vi "Check input.vi"(2 "String to check for":string, 3 "Old table to replace":string[][](table)=[["1", " "], ["2", " "], ["3", " "], ["4", " "], ["5", " "], ["6", " "], ["7", " "], ["8", " "], ["9", " "]]) -> (0 "Guess is correct?":bool, 1 "Output table":string[][](table)=[["1", " "], ["2", " "], ["3", " "], ["4", " "], ["5", " "], ["6", " "], ["7", " "], ["8", " "], ["9", " "]])   [LabVIEW 2023]
panel:
  in  "Answer array":string[](array[string])=["Bulbasaur", "Ivysaur", "Venusaur", "Charmander", "Charmeleon", "Charizard", "Squirtle", "Wartortle", "Blastoise"]
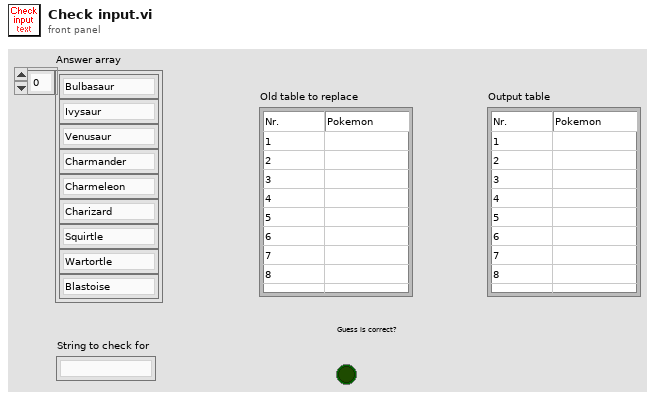
[diagram p1: front panel]
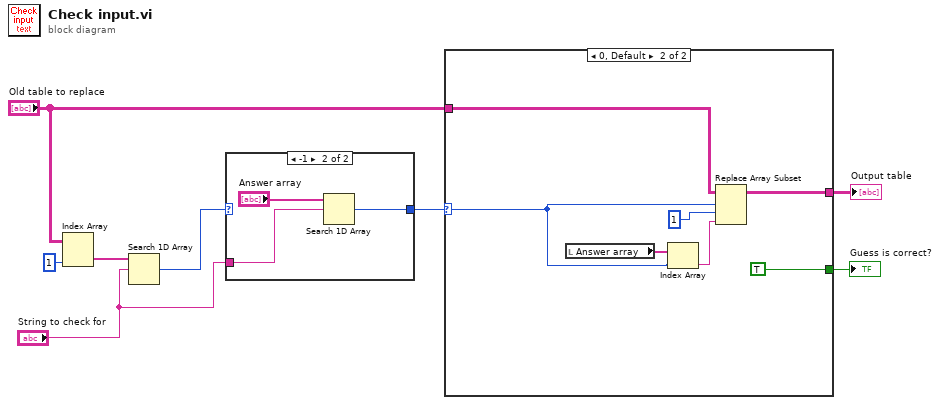
[diagram p0: block diagram]
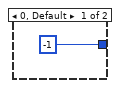
[diagram p2: hidden frame]
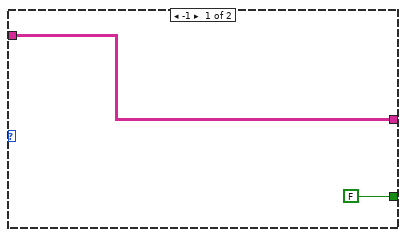
[diagram p3: hidden frame]
diagram:
  n1 = Index Array "Index Array"(array="Old table to replace", index (col)=1 ("index (row)")) -> (element=w2:string[])  [unwired: 1 in]
  n2 = Search 1D Array(1D array=w2, element="String to check for") -> (index of element=w4:i32)  [unwired: 1 in]
  n3 = case shown="-1" w4 {
    tunnel: [-1 ("index of element") w12] -> w3
    tunnel: "String to check for" -> [_ w11]
    frame 0, Default {
    }
    frame -1 {
      n4 = Search 1D Array(1D array="Answer array", element=w11) -> (index of element=w12:i32)  [unwired: 1 in]
    }
  }
  n5 = case shown="0, Default" w3 {
    selector: w3 -> [_ w19]
    tunnel: [w14 w21] -> w8
    tunnel: "Old table to replace" -> [w14 w16]
    tunnel: [FALSE ("Is in array") TRUE ("Is in array")] -> w7
    frame -1 {
    }
    frame 0, Default {
      n6 = local read "Answer array"() -> (w18:string[])
      n7 = Index Array "Index Array"(array=w18, index=w19) -> (element=w17:string)
      n8 = Replace Array Subset "Replace Array Subset"(array=w16, new element=w17, index (row)=w19, index (col)=1 ("disabled index (col)")) -> (w21:string[][])
    }
  }
  "Output table" <- w8
  "Guess is correct?" <- w7
